vi "一体站流程质控自动启动.vi"(6 "CODMn量程切换":enum32{"H", "L", "AUTO"}(ring)=enum."AUTO", 8 "总磷量程切换":enum32{"H", "L", "AUTO"}(ring)=enum."AUTO", 9 "总氮量程切换":enum32{"H", "L", "AUTO"}(ring)=enum."AUTO", 10 "氨氮量程切换":enum32{"H", "L", "AUTO"}(ring)=enum."AUTO", 11 "参数":T1={"是否启用仪器"=FALSE, "CODMn"={"启动测量模式"={"测量模式"=enum."水样测量"}, "确定按钮"=TRUE}, "启动模块"={"氨氮"=FALSE, "总磷"=FALSE, "总氮"=FALSE, "CODMn"=FALSE, "CODCr"=FALSE}, "常规启动"=FALSE, "直接启动"=FALSE}) -> ()   [LabVIEW 2016, in "质控单元.lvlib"]
panel:
  out "枚举 2":enum16{"初始化", "采配水启动", "等待", "配水", "排水", "结束"}(ring)
  out "枚举":enum16{"初始化", "采配水启动", "等待", "配水", "排水", "结束"}(ring)
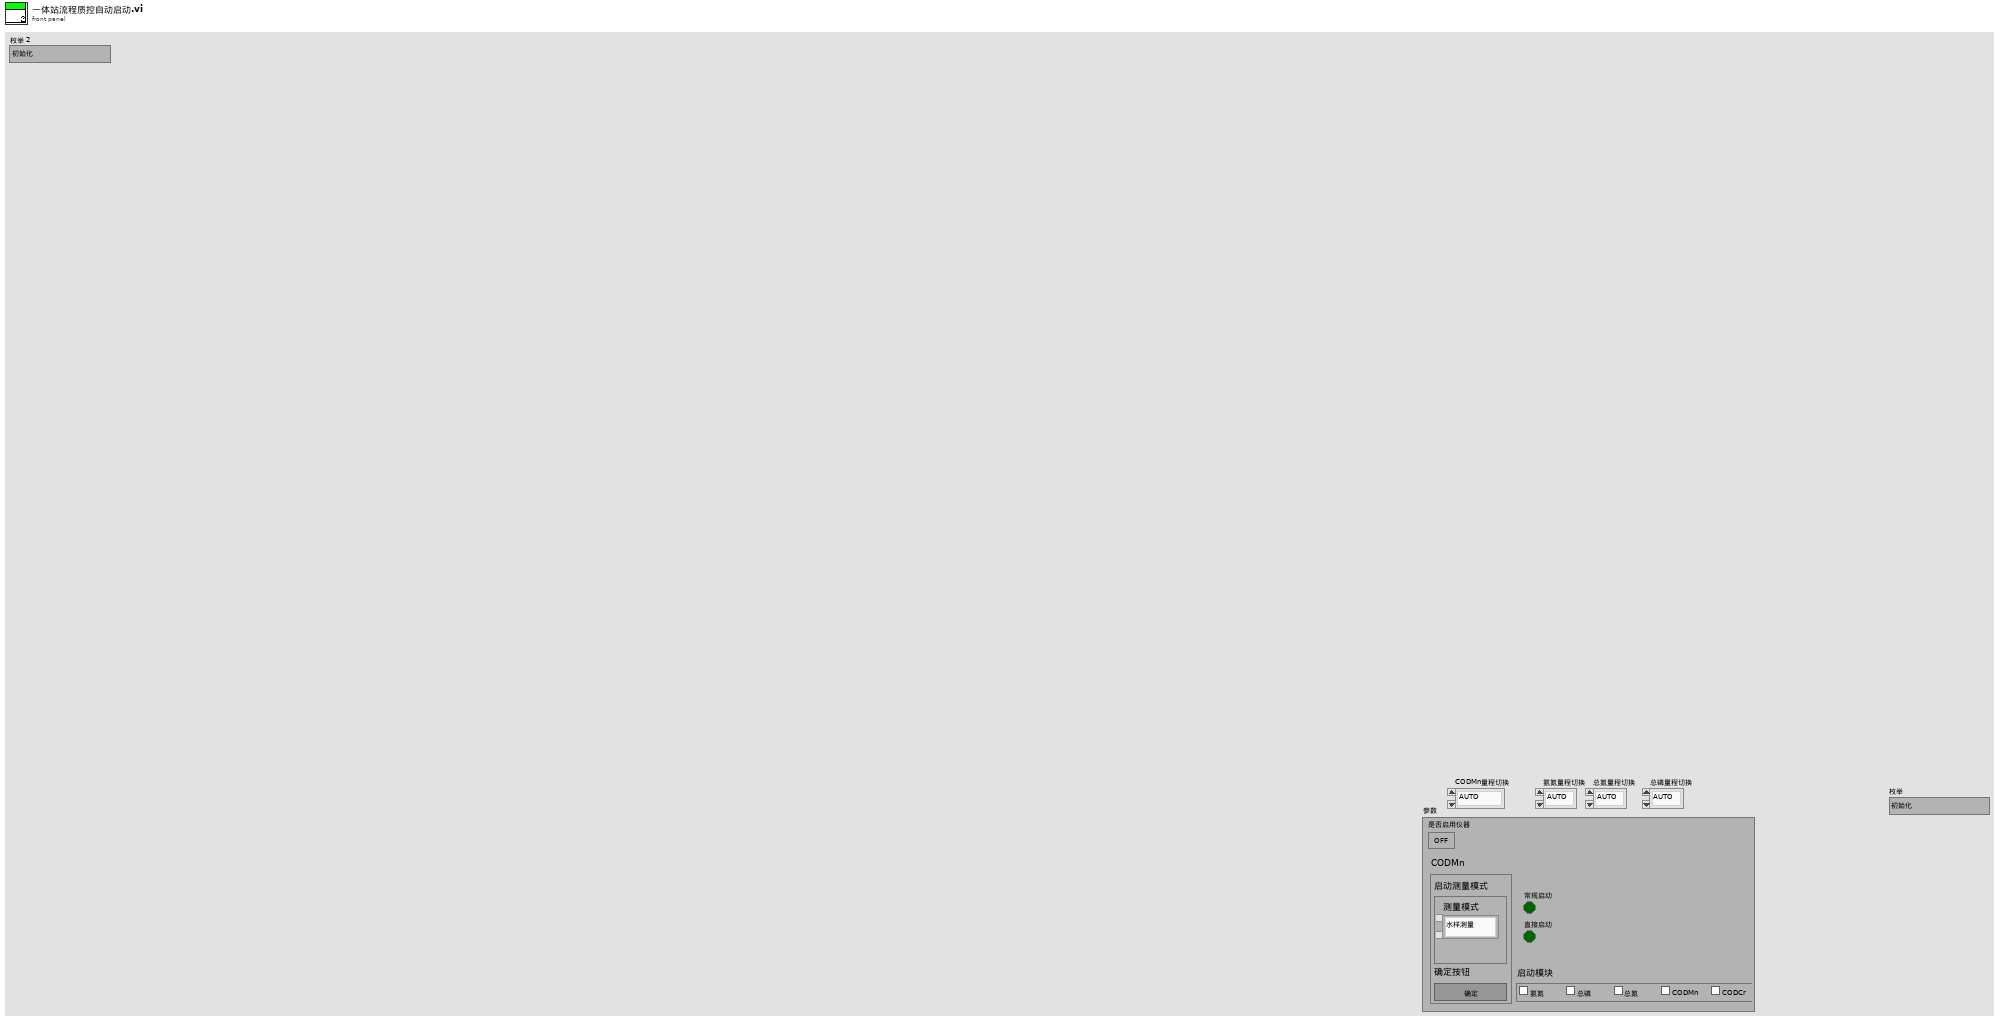
[diagram p1: front panel]
types:
  T1 = cluster{"是否启用仪器":bool, "CODMn":cluster{"启动测量模式":cluster{"测量模式":enum16{"水样测量", "标样核查", "加标回收", "平行样", "校零", "校标"}}, "确定按钮":bool}, "启动模块":cluster{"氨氮":bool, "总磷":bool, "总氮":bool, "CODMn":bool, "CODCr":bool}, "常规启动":bool, "直接启动":bool}
  T2 = cluster{"命令":string, cluster{"starting address":u16, "holding register value":u16}}
  T3 = cluster{"R0":i16, "R1":i16, "R2":i16, "R3":i16, "R4":i16, "R5":i16, "R6":i16, "R7":i16, "R8":i16, "R9":i16, "R10":i16, "R11":i16, "R12":i16, "R13":i16, "R14":i16, "R15":i16, "R16":i16, "R17":i16, "R18":i16, "R19":i16, "R20":i16, "R21":i16, "R22":i16, "R23":i16, "R24":i16, "R25":i16, "R26":i16, "R27":i16, "R28":i16, "R29":i16, "R30":i16, "R31":i16, "R32":i16, "R33":i16, "R34":i16, "R35":i16, "R36":i16, "R37":i16, "R38":i16, "R39":i16, "R40":i16, "R41":i16, "R42":i16, "R43":i16, "R44":i16, "R45":i16, "R46":i16, "R47":i16, "R48":i16, "R49":i16, "R50":i16, "R51":i16, "R52":i16, "R53":i16, "R54":i16, "R55":i16, "R56":i16}
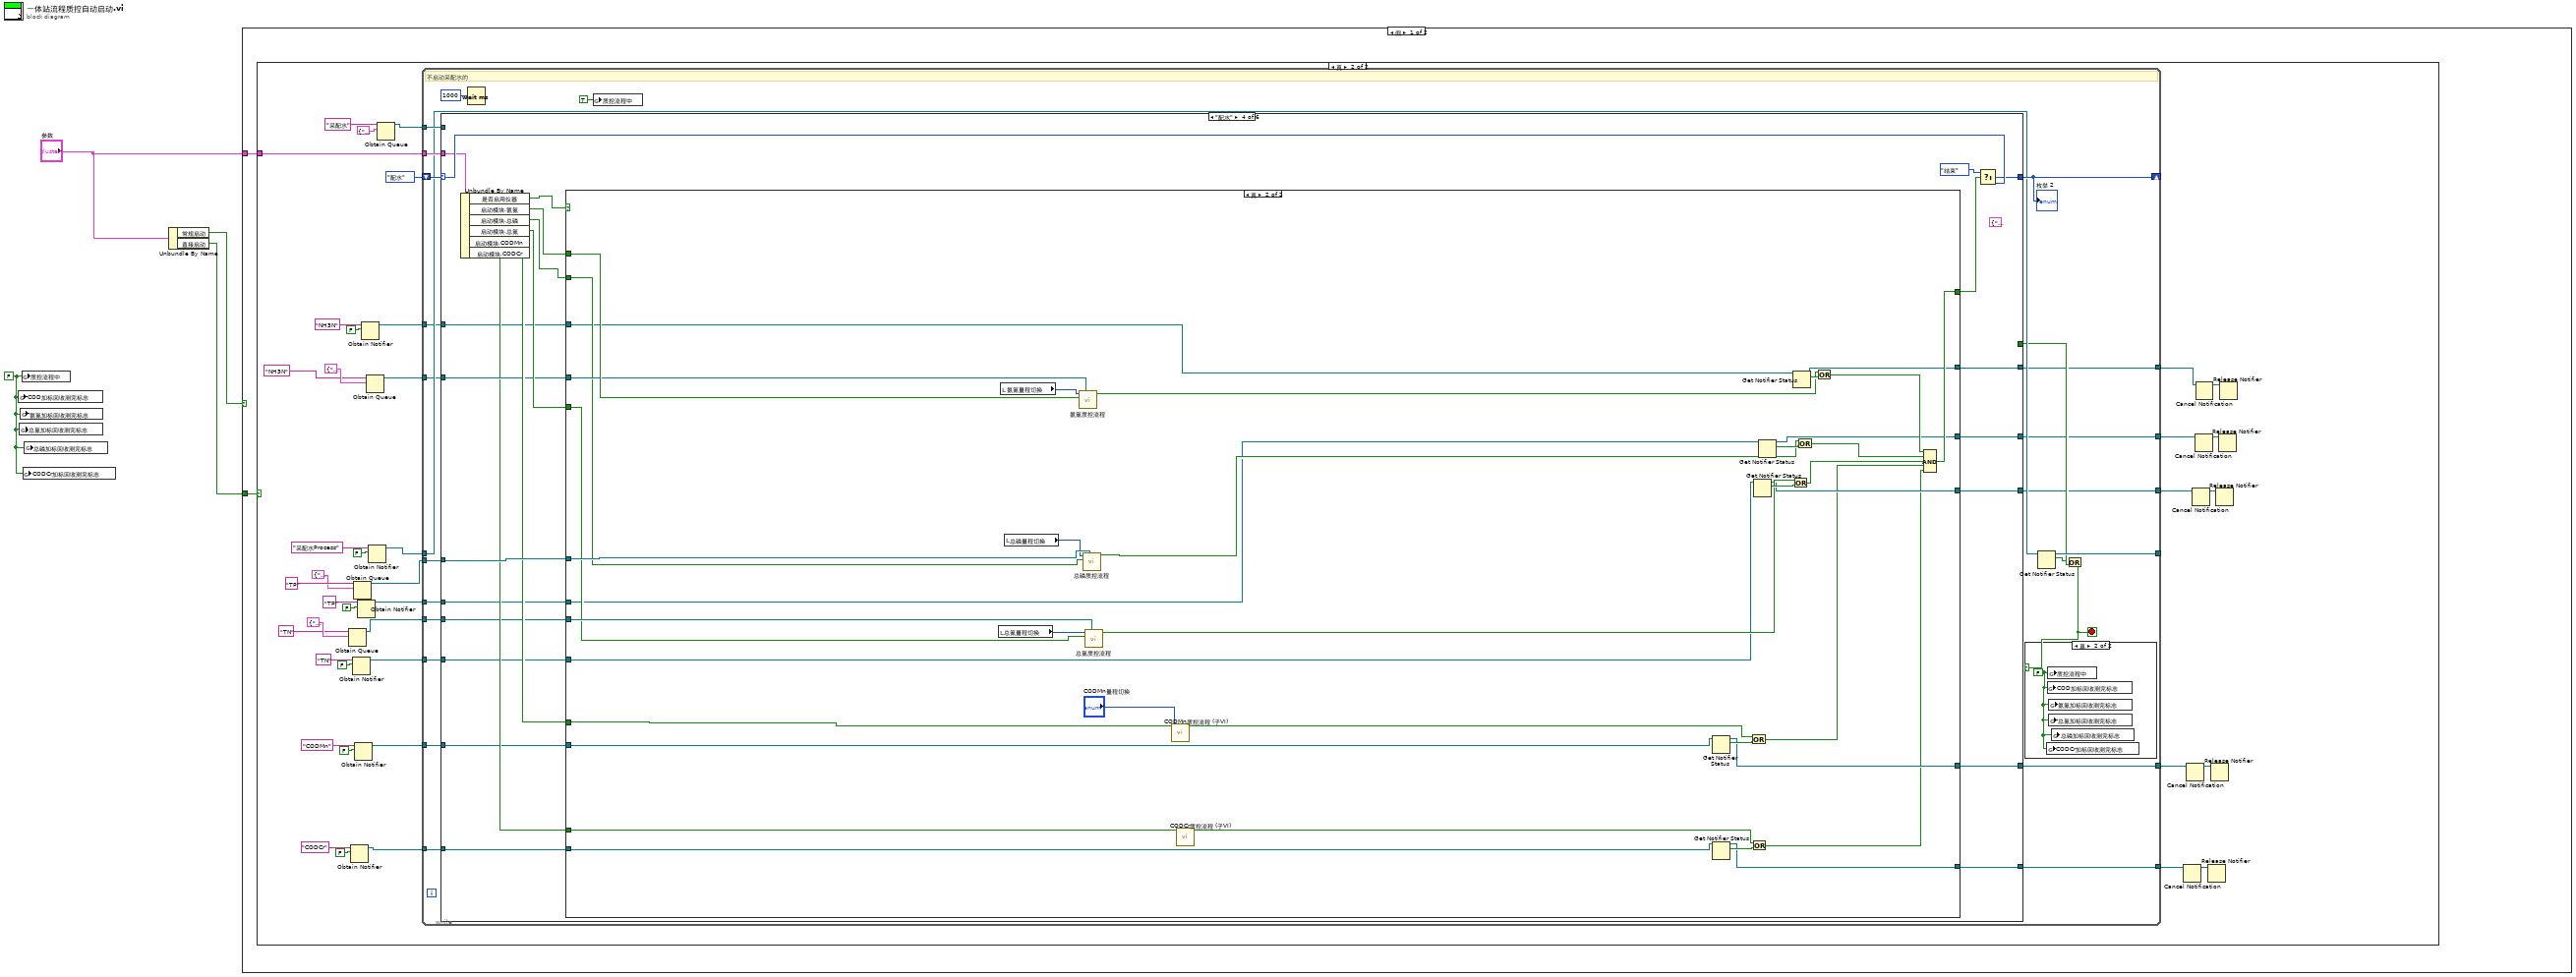
[diagram p0: block diagram]
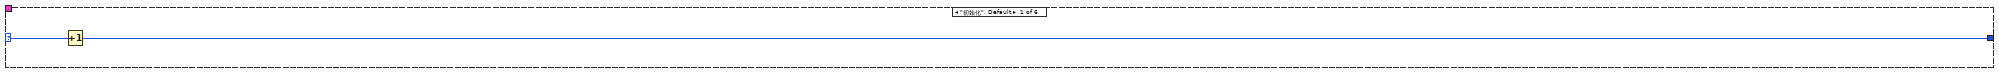
[diagram p4: hidden frame]
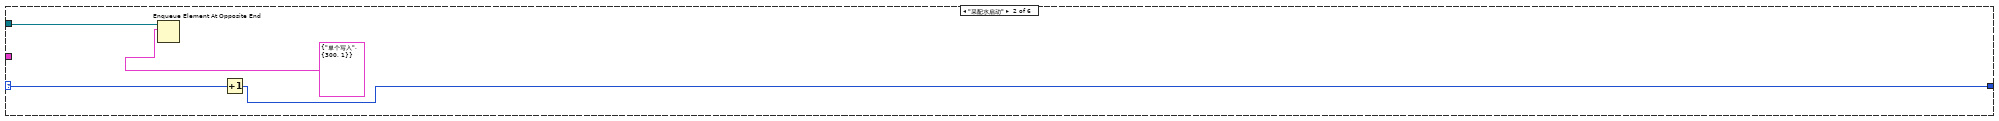
[diagram p5: hidden frame]
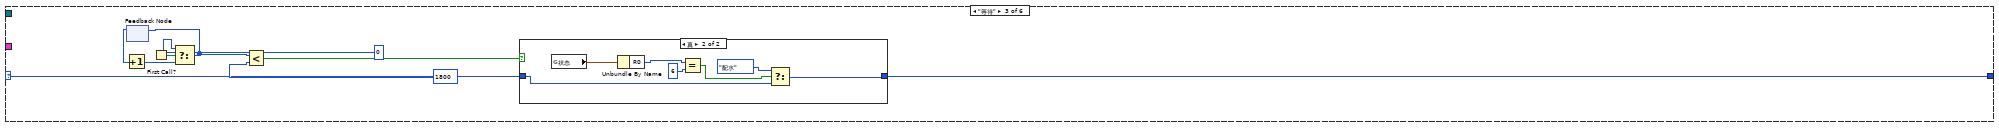
[diagram p6: hidden frame]
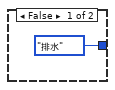
[diagram p7: hidden frame]
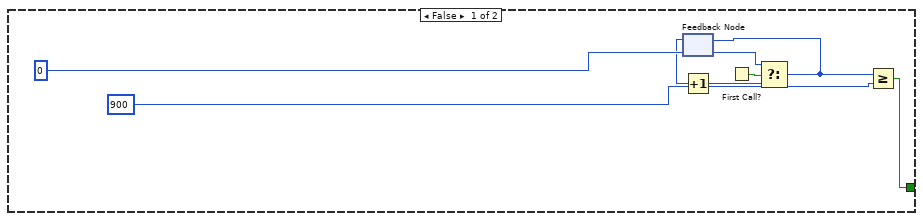
[diagram p8: hidden frame]
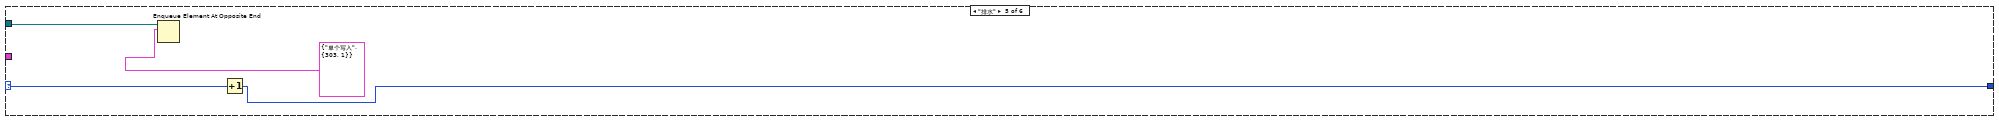
[diagram p9: hidden frame]
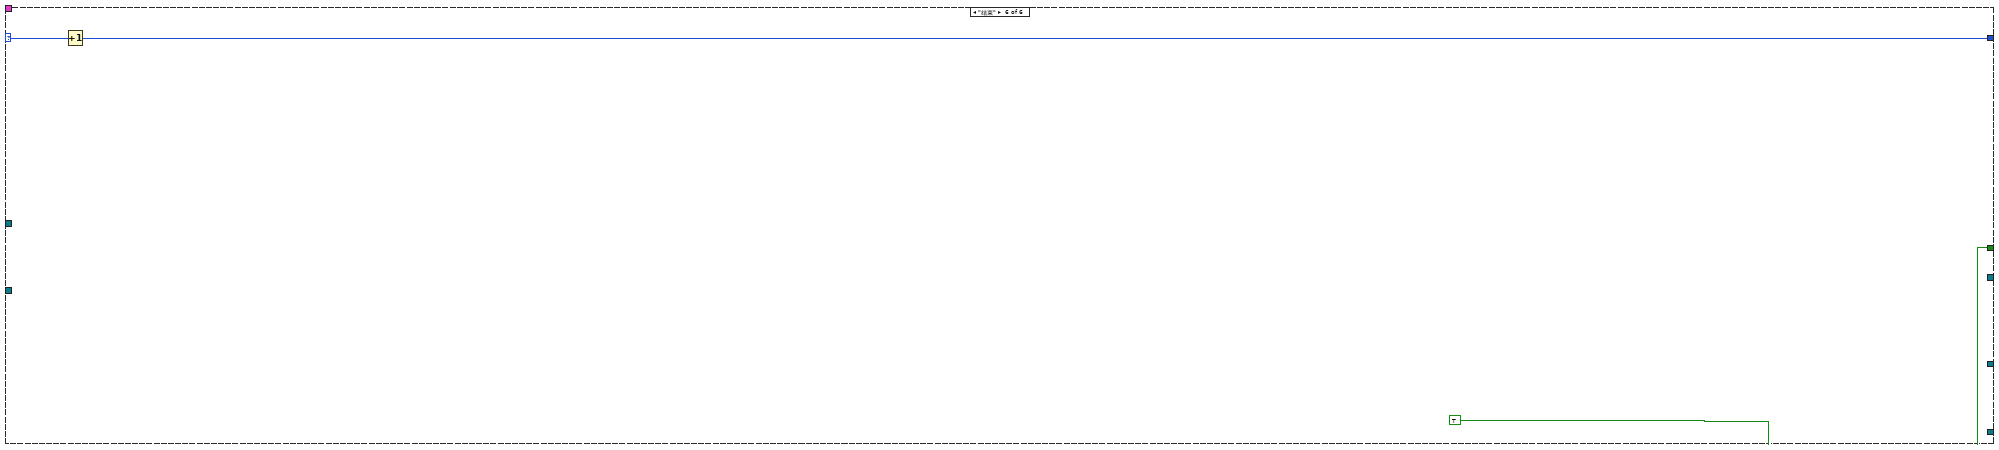
[diagram p10: hidden frame]
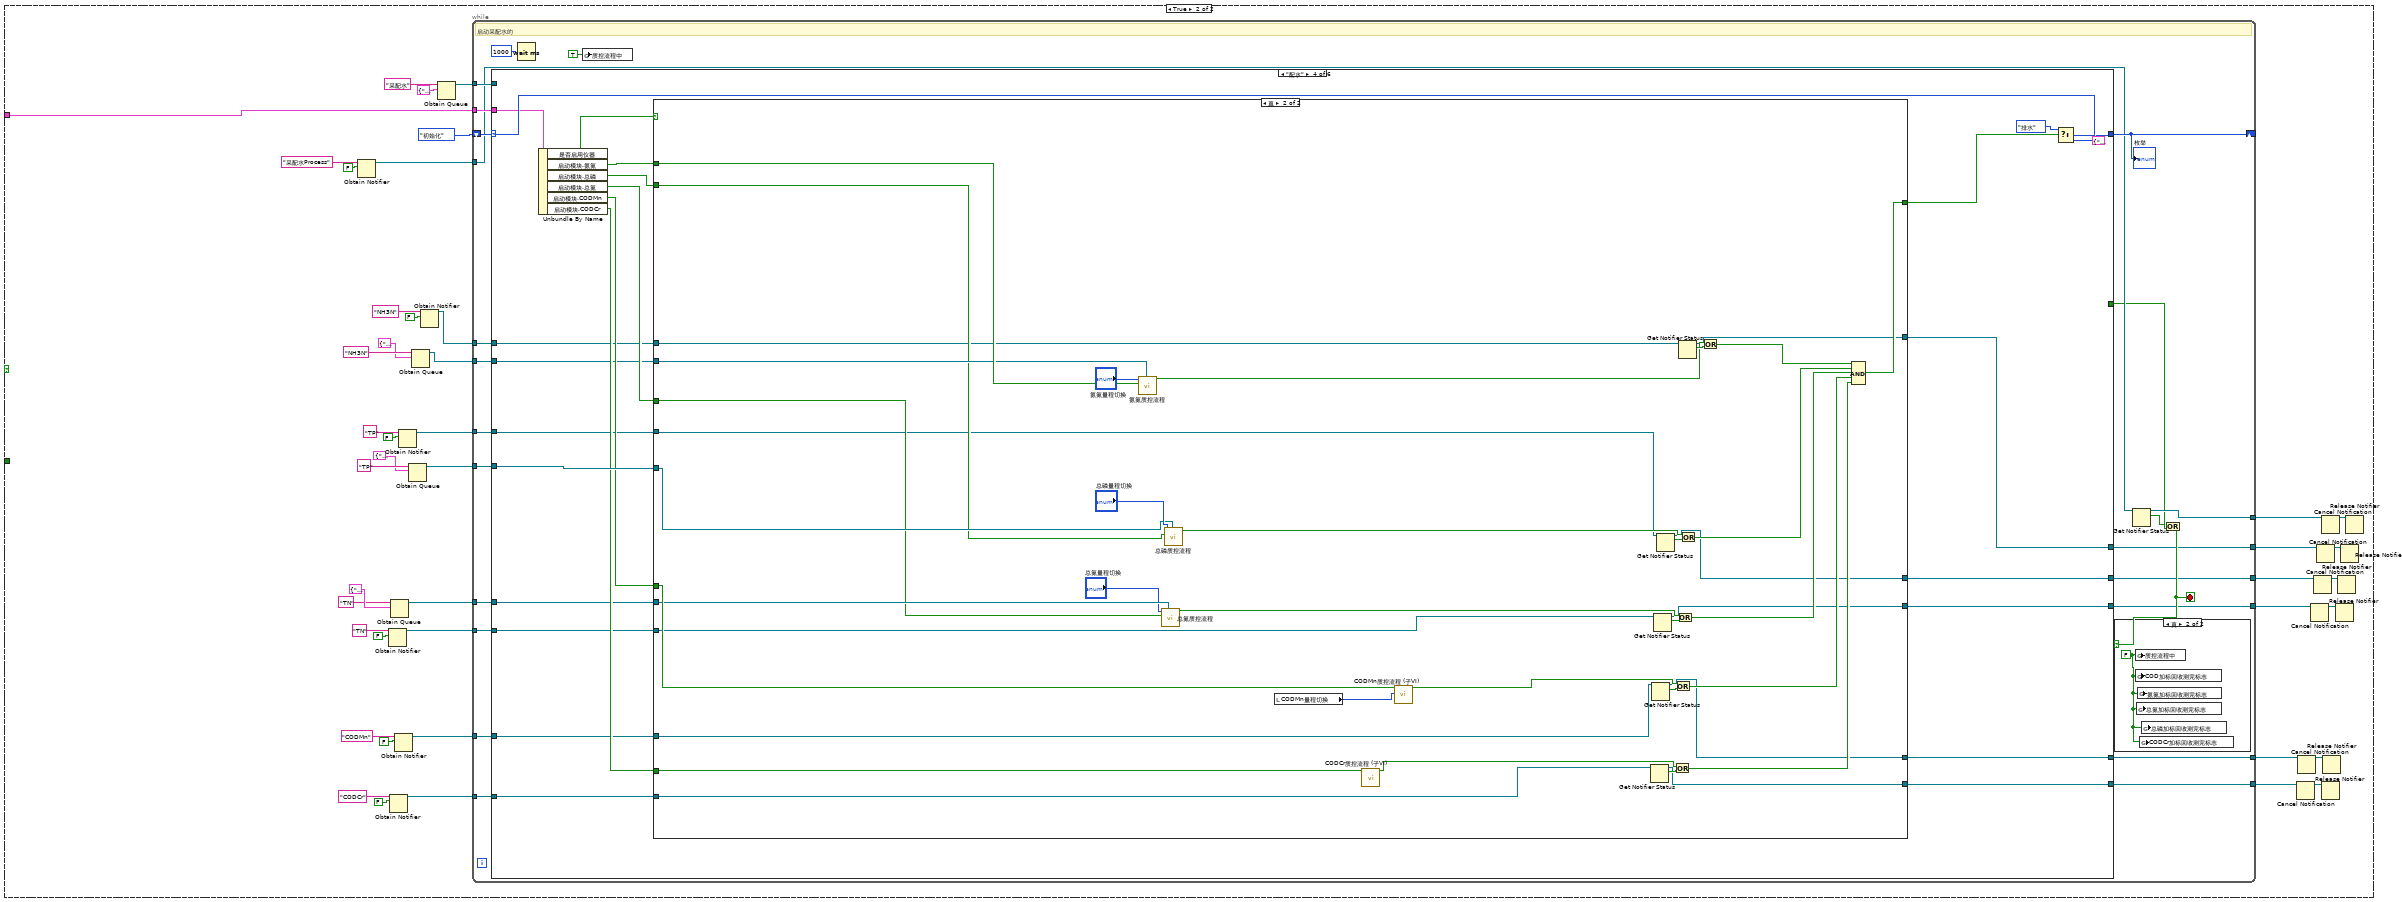
[diagram p11: hidden frame]
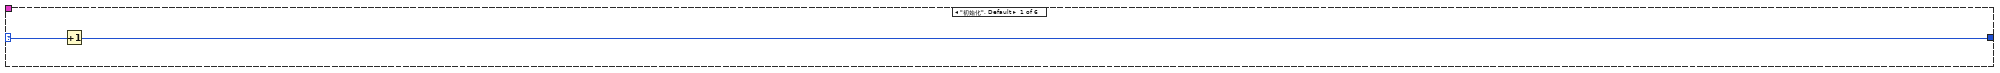
[diagram p13: hidden frame]
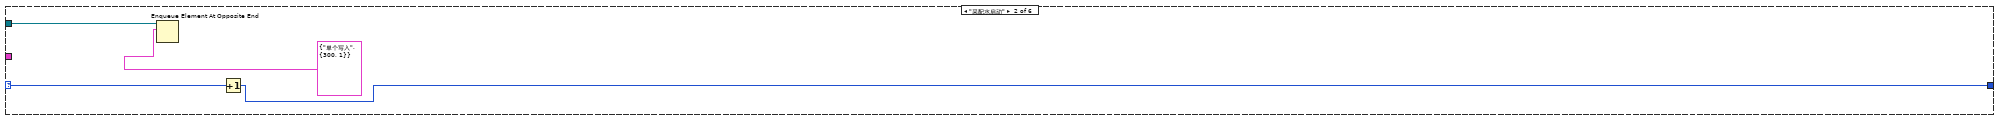
[diagram p14: hidden frame]
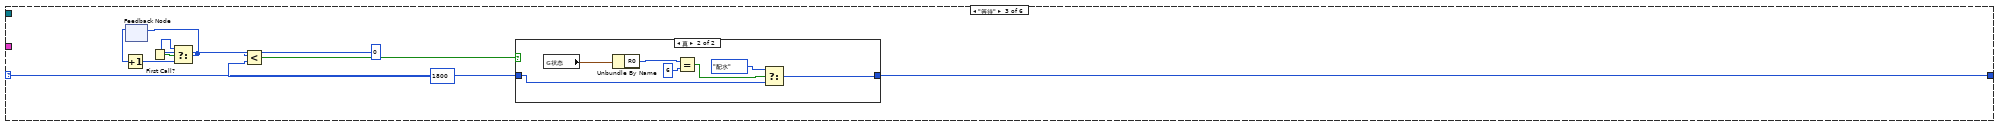
[diagram p15: hidden frame]
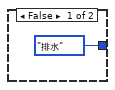
[diagram p16: hidden frame]
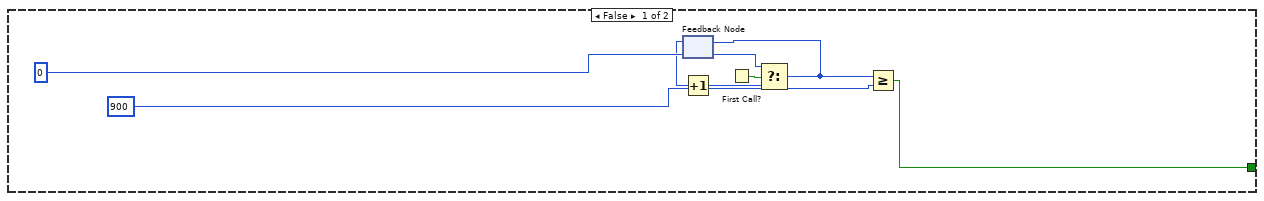
[diagram p17: hidden frame]
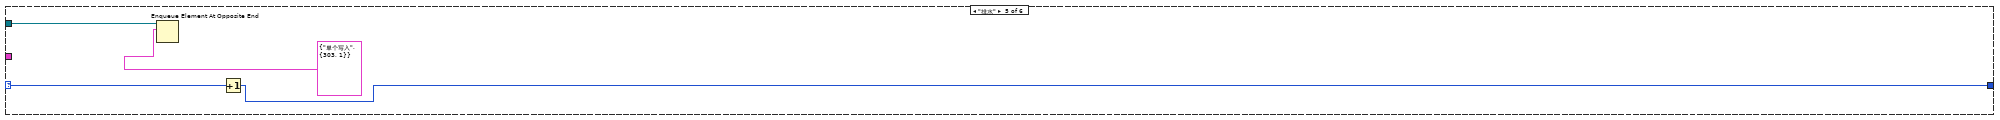
[diagram p18: hidden frame]
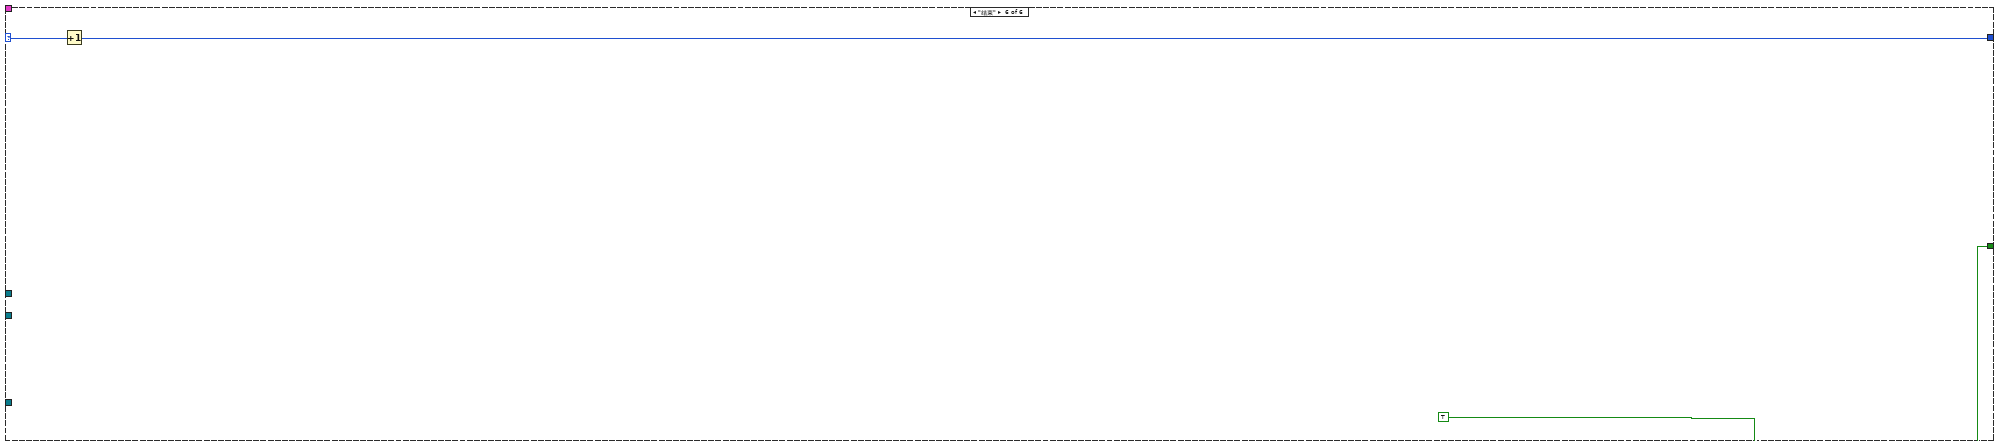
[diagram p19: hidden frame]
diagram:
  w1 = FALSE ("质控流程中")
  n1 = global write "质控测完标志全局 1.vi" "COD加标回收测完标志"(w1) -> ()
  n2 = global write "质控测完标志全局 1.vi" "总氮加标回收测完标志"(w1) -> ()
  n3 = global write "质控测完标志全局 1.vi" "氨氮加标回收测完标志"(w1) -> ()
  n4 = global write "质控测完标志全局 1.vi" "质控流程中"(w1) -> ()
  n5 = global write "质控测完标志全局 1.vi" "CODCr加标回收测完标志"(w1) -> ()
  n6 = global write "质控测完标志全局 1.vi" "总磷加标回收测完标志"(w1) -> ()
  n7 = Unbundle By Name("参数") -> ("常规启动"=w3:bool, "直接启动"=w2:bool)
  n8 = case shown="假" w3 {
    tunnel: "参数" -> [w5 w204]
    tunnel: w2 -> [w6 _]
    frame False {
      n9 = case shown="真" w6 {
        tunnel: w5 -> [_ w47]
        frame False {
        }
        frame True {
          n10 = Obtain Queue(name (unnamed)="TN" ("名称（未命名）"), element data type=cluster{"命令":string, "data":variant} {"命令"="", "data"=variant}) -> (queue out=w32:refnum<queue>)  [unwired: 3 in, 2 out]
          n11 = Obtain Notifier(name (unnamed)="CODCr" ("名称（未命名）"), notification data type=FALSE) -> (notifier out=w9:refnum<notifier>)  [unwired: 2 in, 2 out]
          n12 = Obtain Notifier(name (unnamed)="TN" ("名称（未命名）"), notification data type=FALSE) -> (notifier out=w15:refnum<notifier>)  [unwired: 2 in, 2 out]
          n13 = Obtain Queue(name (unnamed)="TP" ("名称（未命名）"), element data type=cluster{"命令":string, "data":variant} {"命令"="", "data"=variant}) -> (queue out=w38:refnum<queue>)  [unwired: 3 in, 2 out]
          n14 = Obtain Notifier(name (unnamed)="CODMn" ("名称（未命名）"), notification data type=FALSE) -> (notifier out=w12:refnum<notifier>)  [unwired: 2 in, 2 out]
          n15 = Obtain Notifier(name (unnamed)="TP" ("名称（未命名）"), notification data type=FALSE) -> (notifier out=w18:refnum<notifier>)  [unwired: 2 in, 2 out]
          n16 = Obtain Notifier(name (unnamed)="NH3N" ("名称（未命名）"), notification data type=FALSE) -> (notifier out=w21:refnum<notifier>)  [unwired: 2 in, 2 out]
          n17 = Obtain Queue(name (unnamed)="NH3N" ("名称（未命名）"), element data type=cluster{"命令":string, "data":variant} {"命令"="", "data"=variant}) -> (queue out=w35:refnum<queue>)  [unwired: 3 in, 2 out]
          n18 = Obtain Notifier(name (unnamed)="采配水Process" ("名称（未命名）"), notification data type=FALSE) -> (notifier out=w41:refnum<notifier>)  [unwired: 2 in, 2 out]
          n19 = Obtain Queue(name (unnamed)="采配水" ("名称（未命名）"), element data type=cluster{"命令":string, "数据":variant} {"命令"="", "数据"=variant}) -> (queue out=w44:refnum<queue>)  [unwired: 3 in, 2 out]
          n20 = while {
            tunnel: w44 -> [w72]
            shift-right: [w70] -> _
            shift-left: enum16{"初始化", "采配水启动", "等待", "配水", "排水", "结束"}."配水" ("枚举") -> [w71]
            tunnel: w38 -> [w68]
            tunnel: w47 -> [w67]
            tunnel: w41 -> [w66]
            tunnel: [w65] -> _
            tunnel: w35 -> [w62]
            tunnel: w32 -> [w59]
            tunnel: w21 -> [w58]
            tunnel: [w57] -> w19
            tunnel: w18 -> [w56]
            tunnel: [w55] -> w16
            tunnel: w15 -> [w54]
            tunnel: [w53] -> w13
            tunnel: w12 -> [w52]
            tunnel: [w51] -> w10
            tunnel: w9 -> [w50]
            tunnel: [w49] -> w7
            stop <- w61 stop-if-true
            # "不启动采配水的"
            n21 = case shown="\"配水\"" w71 {
              selector: w71 -> [w75 w77 w86 w119 w167 w172]
              tunnel: w72 -> [_ w78 _ _ w168 _]
              tunnel: [w74 w76 w85 w118 w166 w171] -> w70
              tunnel: [_ _ _ _ _ TRUE] -> w64
              tunnel: w68 -> [_ _ _ w117 _ _]
              tunnel: w67 -> [_ _ _ w114 _ _]
              tunnel: w62 -> [_ _ _ w109 _ _]
              tunnel: w59 -> [_ _ _ w107 _ _]
              tunnel: w58 -> [_ _ _ w106 _ _]
              tunnel: [_ _ _ w105 _ _] -> w57
              tunnel: w56 -> [_ _ _ w104 _ _]
              tunnel: [_ _ _ w103 _ _] -> w55
              tunnel: w54 -> [_ _ _ w102 _ _]
              tunnel: [_ _ _ w101 _ _] -> w53
              tunnel: w52 -> [_ _ _ w100 _ _]
              tunnel: [_ _ _ w99 _ _] -> w51
              tunnel: w50 -> [_ _ _ w98 _ _]
              tunnel: [_ _ _ w97 _ _] -> w49
              frame "初始化", Default {
                n22 = Increment(x=w75) -> (x+1=w74:enum16{"初始化", "采配水启动", "等待", "配水", "排水", "结束"})
              }
              frame "采配水启动" {
                n23 = Enqueue Element At Opposite End(queue=w78, element=T2 {"命令"="单个写入", {"starting address"=300, "holding register value"=1}} ("元素")) -> ()  [unwired: 2 in, 3 out]
                n24 = Increment(x=w77) -> (x+1=w76:enum16{"初始化", "采配水启动", "等待", "配水", "排水", "结束"})
              }
              frame "等待" {
                n25 = feedback #1() -> (w82:i32)  [unwired: 1 in]
                n26 = Increment(x=w82) -> (x+1=w81:i32)
                n27 = First Call?() -> (First Call?: T/F=w83:bool)
                n28 = Select(t=0, s=w83, f=w81) -> (s? t:f=w80:i32)
                n29 = feedback-in #1(w80) -> ()
                n30 = Less?(x=w80, y=1800) -> (x < y?=w87:bool)
                n31 = case shown="真" w87 {
                  tunnel: w86 -> [_ w92]
                  tunnel: [enum16{"初始化", "采配水启动", "等待", "配水", "排水", "结束"}."排水" ("枚举") w91] -> w85
                  frame False {
                  }
                  frame True {
                    n32 = global read "与采配水交互全局.vi" "状态"() -> (w90:T3)
                    n33 = Unbundle By Name(w90) -> ("R0"=w96:i16)
                    n34 = Equal?(x=w96, y=i16 6) -> (x = y?=w94:bool)
                    n35 = Select(t=enum16{"初始化", "采配水启动", "等待", "配水", "排水", "结束"}."配水" ("枚举"), s=w94, f=w92) -> (s? t:f=w91:enum16{"初始化", "采配水启动", "等待", "配水", "排水", "结束"})
                  }
                }
              }
              frame "配水" {
                (unwired) cluster{"命令":string, "data":variant} {"命令"="启动", "data"=variant(cluster{"站号":u16, "控制命令输出":u16[]} {"站号"=1, "控制命令输出"=[256, 0]})} ("元素")
                n36 = Unbundle By Name(w114) -> ("是否启用仪器"=w116:bool, "启动模块.氨氮"=w112:bool, "启动模块.总磷"=w113:bool, "启动模块.总氮"=w110:bool, "启动模块.CODMn"=w111:bool, "启动模块.CODCr"=w108:bool)
                n37 = case shown="真" w116 {
                  tunnel: w117 -> [_ w158]
                  tunnel: [w121 w165] -> w115
                  tunnel: w113 -> [_ w156]
                  tunnel: w112 -> [_ w164]
                  tunnel: w111 -> [_ w163]
                  tunnel: w110 -> [_ w153]
                  tunnel: w109 -> [_ w162]
                  tunnel: w108 -> [_ w159]
                  tunnel: w107 -> [_ w155]
                  tunnel: w106 -> [_ w149]
                  tunnel: [_ w148] -> w105
                  tunnel: w104 -> [_ w145]
                  tunnel: [_ w143] -> w103
                  tunnel: w102 -> [_ w140]
                  tunnel: [_ w138] -> w101
                  tunnel: w100 -> [_ w134]
                  tunnel: [_ w133] -> w99
                  tunnel: w98 -> [_ w129]
                  tunnel: [_ w128] -> w97
                  frame False {
                    n38 = feedback #2() -> (w125:i32)  [unwired: 1 in]
                    n39 = Increment(x=w125) -> (x+1=w124:i32)
                    n40 = First Call?() -> (First Call?: T/F=w126:bool)
                    n41 = Select(t=0, s=w126, f=w124) -> (s? t:f=w122:i32)
                    n42 = feedback-in #2(w122) -> ()
                    n43 = Greater Or Equal?(x=w122, y=900) -> (x >= y?=w121:bool)
                  }
                  frame True {
                    n44 = local read "总氮量程切换"() -> (w154:enum32{"H", "L", "AUTO"})
                    n45 = local read "氨氮量程切换"() -> (w160:enum32{"H", "L", "AUTO"})
                    n46 = local read "总磷量程切换"() -> (w157:enum32{"H", "L", "AUTO"})
                    n47 = call "氨氮质控流程.vi"("队列输入NH3"=w162, "氨氮"=w164, "氨氮量程切换"=w160) -> ("布尔"=w150:bool)  [unwired: 7 in]
                    n48 = call "总磷质控流程.vi"("队列输入TP"=w158, "总磷"=w156, "总磷量程切换"=w157) -> ("布尔"=w146:bool)  [unwired: 7 in]
                    n49 = call "总氮质控流程.vi"("队列输入TN"=w155, "总氮"=w153, "总氮量程切换"=w154) -> ("布尔"=w141:bool)  [unwired: 7 in]
                    n50 = call "CODMn质控流程 (子VI).vi"("CODMn量程切换"="CODMn量程切换", "CODMn"=w163) -> ("布尔"=w136:bool)  [unwired: 8 in]
                    n51 = call "CODCr质控流程 (子VI).vi"("CODCr"=w159) -> ("布尔"=w131:bool)  [unwired: 9 in]
                    n52 = Get Notifier Status(notifier=w134) -> (notifier out=w133:refnum<notifier>, current notification=w137:bool)  [unwired: 1 in, 3 out]
                    n53 = Get Notifier Status(notifier=w129) -> (notifier out=w128:refnum<notifier>, current notification=w132:bool)  [unwired: 1 in, 3 out]
                    n54 = Or(x=w136, y=w137) -> (x .or. y?=w135:bool)
                    n55 = Or(x=w131, y=w132) -> (x .or. y?=w130:bool)
                    n56 = Get Notifier Status(notifier=w140) -> (notifier out=w138:refnum<notifier>, current notification=w142:bool)  [unwired: 1 in, 3 out]
                    n57 = Get Notifier Status(notifier=w145) -> (notifier out=w143:refnum<notifier>, current notification=w147:bool)  [unwired: 1 in, 3 out]
                    n58 = Or(x=w141, y=w142) -> (x .or. y?=w139:bool)
                    n59 = Get Notifier Status(notifier=w149) -> (notifier out=w148:refnum<notifier>, current notification=w152:bool)  [unwired: 1 in, 3 out]
                    n60 = Or(x=w146, y=w147) -> (x .or. y?=w144:bool)
                    n61 = Or(x=w150, y=w152) -> (x .or. y?=w151:bool)
                    n62 = Compound Arithmetic op=AND ("复合运算")(w151, w144, w139, w135, w130) -> (w165:bool)
                  }
                }
                n63 = Select(t=enum16{"初始化", "采配水启动", "等待", "配水", "排水", "结束"}."结束" ("枚举"), s=w115, f=w119) -> (s? t:f=w118:enum16{"初始化", "采配水启动", "等待", "配水", "排水", "结束"})
              }
              frame "排水" {
                n64 = Enqueue Element At Opposite End(queue=w168, element=T2 {"命令"="单个写入", {"starting address"=303, "holding register value"=1}} ("元素")) -> ()  [unwired: 2 in, 3 out]
                n65 = Increment(x=w167) -> (x+1=w166:enum16{"初始化", "采配水启动", "等待", "配水", "排水", "结束"})
              }
              frame "结束" {
                n66 = Increment(x=w172) -> (x+1=w171:enum16{"初始化", "采配水启动", "等待", "配水", "排水", "结束"})
              }
            }
            "枚举 2" <- w70
            n67 = Wait (ms)(milliseconds to wait=u32 1000 ("等待时间（毫秒）")) -> ()  [unwired: 1 out]
            n68 = global write "质控测完标志全局 1.vi" "质控流程中"(TRUE ("质控流程中")) -> ()
            n69 = Get Notifier Status(notifier=w66) -> (notifier out=w65:refnum<notifier>, current notification=w63:bool)  [unwired: 1 in, 3 out]
            n70 = Or(x=w63, y=w64) -> (x .or. y?=w61:bool)
            n71 = case shown="真" w61 {
              frame False {
              }
              frame True {
                w73 = FALSE ("质控流程中")
                n72 = global write "质控测完标志全局 1.vi" "CODCr加标回收测完标志"(w73) -> ()
                n73 = global write "质控测完标志全局 1.vi" "COD加标回收测完标志"(w73) -> ()
                n74 = global write "质控测完标志全局 1.vi" "质控流程中"(w73) -> ()
                n75 = global write "质控测完标志全局 1.vi" "总氮加标回收测完标志"(w73) -> ()
                n76 = global write "质控测完标志全局 1.vi" "氨氮加标回收测完标志"(w73) -> ()
                n77 = global write "质控测完标志全局 1.vi" "总磷加标回收测完标志"(w73) -> ()
              }
            }
          }
          n78 = Cancel Notification(0:w7) -> (8:w8:refnum<notifier>)  [unwired: 1 in, 2 out]
          n79 = Cancel Notification(0:w10) -> (8:w11:refnum<notifier>)  [unwired: 1 in, 2 out]
          n80 = Cancel Notification(0:w13) -> (8:w14:refnum<notifier>)  [unwired: 1 in, 2 out]
          n81 = Cancel Notification(0:w16) -> (8:w17:refnum<notifier>)  [unwired: 1 in, 2 out]
          n82 = Cancel Notification(0:w19) -> (8:w20:refnum<notifier>)  [unwired: 1 in, 2 out]
          n83 = Release Notifier(notifier=w8) -> ()  [unwired: 2 in, 3 out]
          n84 = Release Notifier(notifier=w11) -> ()  [unwired: 2 in, 3 out]
          n85 = Release Notifier(notifier=w14) -> ()  [unwired: 2 in, 3 out]
          n86 = Release Notifier(notifier=w17) -> ()  [unwired: 2 in, 3 out]
          n87 = Release Notifier(notifier=w20) -> ()  [unwired: 2 in, 3 out]
        }
      }
    }
    frame True {
      n88 = Obtain Notifier(name (unnamed)="采配水Process" ("名称（未命名）"), notification data type=FALSE) -> (notifier out=w207:refnum<notifier>)  [unwired: 2 in, 2 out]
      n89 = Obtain Notifier(name (unnamed)="TN" ("名称（未命名）"), notification data type=FALSE) -> (notifier out=w189:refnum<notifier>)  [unwired: 2 in, 2 out]
      n90 = Obtain Notifier(name (unnamed)="CODCr" ("名称（未命名）"), notification data type=FALSE) -> (notifier out=w183:refnum<notifier>)  [unwired: 2 in, 2 out]
      n91 = Obtain Queue(name (unnamed)="TN" ("名称（未命名）"), element data type=cluster{"命令":string, "data":variant} {"命令"="", "data"=variant}) -> (queue out=w201:refnum<queue>)  [unwired: 3 in, 2 out]
      n92 = Obtain Notifier(name (unnamed)="CODMn" ("名称（未命名）"), notification data type=FALSE) -> (notifier out=w184:refnum<notifier>)  [unwired: 2 in, 2 out]
      n93 = Obtain Notifier(name (unnamed)="TP" ("名称（未命名）"), notification data type=FALSE) -> (notifier out=w190:refnum<notifier>)  [unwired: 2 in, 2 out]
      n94 = Obtain Queue(name (unnamed)="TP" ("名称（未命名）"), element data type=cluster{"命令":string, "data":variant} {"命令"="", "data"=variant}) -> (queue out=w210:refnum<queue>)  [unwired: 3 in, 2 out]
      n95 = Obtain Queue(name (unnamed)="NH3N" ("名称（未命名）"), element data type=cluster{"命令":string, "data":variant} {"命令"="", "data"=variant}) -> (queue out=w196:refnum<queue>)  [unwired: 3 in, 2 out]
      n96 = Obtain Notifier(name (unnamed)="NH3N" ("名称（未命名）"), notification data type=FALSE) -> (notifier out=w195:refnum<notifier>)  [unwired: 2 in, 2 out]
      n97 = Obtain Queue(name (unnamed)="采配水" ("名称（未命名）"), element data type=cluster{"命令":string, "数据":variant} {"命令"="", "数据"=variant}) -> (queue out=w214:refnum<queue>)  [unwired: 3 in, 2 out]
      n98 = while {
        tunnel: w214 -> [w240]
        shift-right: [w238] -> _
        shift-left: enum16{"初始化", "采配水启动", "等待", "配水", "排水", "结束"}."初始化" ("枚举") -> [w239]
        tunnel: w210 -> [w236]
        tunnel: w204 -> [w235]
        tunnel: w207 -> [w234]
        tunnel: [w233] -> w206
        tunnel: w201 -> [w228]
        tunnel: w196 -> [w227]
        tunnel: w195 -> [w226]
        tunnel: w190 -> [w225]
        tunnel: w189 -> [w224]
        tunnel: w184 -> [w223]
        tunnel: w183 -> [w222]
        tunnel: [w221] -> w181
        tunnel: [w220] -> w179
        tunnel: [w219] -> w177
        tunnel: [w218] -> w175
        tunnel: [w217] -> w173
        stop <- w230 stop-if-true
        # "启动采配水的"
        n99 = case shown="\"配水\"" w239 {
          selector: w239 -> [w243 w245 w254 w287 w335 w340]
          tunnel: w240 -> [_ w246 _ _ w336 _]
          tunnel: [w242 w244 w253 w286 w334 w339] -> w238
          tunnel: [_ _ _ _ _ TRUE] -> w232
          tunnel: w236 -> [_ _ _ w285 _ _]
          tunnel: w235 -> [_ _ _ w282 _ _]
          tunnel: w228 -> [_ _ _ w276 _ _]
          tunnel: w227 -> [_ _ _ w275 _ _]
          tunnel: w226 -> [_ _ _ w274 _ _]
          tunnel: w225 -> [_ _ _ w273 _ _]
          tunnel: w224 -> [_ _ _ w272 _ _]
          tunnel: w223 -> [_ _ _ w271 _ _]
          tunnel: w222 -> [_ _ _ w270 _ _]
          tunnel: [_ _ _ w269 _ _] -> w221
          tunnel: [_ _ _ w268 _ _] -> w220
          tunnel: [_ _ _ w267 _ _] -> w219
          tunnel: [_ _ _ w266 _ _] -> w218
          tunnel: [_ _ _ w265 _ _] -> w217
          frame "初始化", Default {
            n100 = Increment(x=w243) -> (x+1=w242:enum16{"初始化", "采配水启动", "等待", "配水", "排水", "结束"})
          }
          frame "采配水启动" {
            n101 = Enqueue Element At Opposite End(queue=w246, element=T2 {"命令"="单个写入", {"starting address"=300, "holding register value"=1}} ("元素")) -> ()  [unwired: 2 in, 3 out]
            n102 = Increment(x=w245) -> (x+1=w244:enum16{"初始化", "采配水启动", "等待", "配水", "排水", "结束"})
          }
          frame "等待" {
            n103 = feedback #3() -> (w250:i32)  [unwired: 1 in]
            n104 = Increment(x=w250) -> (x+1=w249:i32)
            n105 = First Call?() -> (First Call?: T/F=w251:bool)
            n106 = Select(t=0, s=w251, f=w249) -> (s? t:f=w248:i32)
            n107 = feedback-in #3(w248) -> ()
            n108 = Less?(x=w248, y=1800) -> (x < y?=w255:bool)
            n109 = case shown="真" w255 {
              tunnel: w254 -> [_ w260]
              tunnel: [enum16{"初始化", "采配水启动", "等待", "配水", "排水", "结束"}."排水" ("枚举") w259] -> w253
              frame False {
              }
              frame True {
                n110 = global read "与采配水交互全局.vi" "状态"() -> (w258:T3)
                n111 = Unbundle By Name(w258) -> ("R0"=w264:i16)
                n112 = Equal?(x=w264, y=i16 6) -> (x = y?=w262:bool)
                n113 = Select(t=enum16{"初始化", "采配水启动", "等待", "配水", "排水", "结束"}."配水" ("枚举"), s=w262, f=w260) -> (s? t:f=w259:enum16{"初始化", "采配水启动", "等待", "配水", "排水", "结束"})
              }
            }
          }
          frame "配水" {
            (unwired) cluster{"命令":string, "data":variant} {"命令"="启动", "data"=variant(cluster{"站号":u16, "控制命令输出":u16[]} {"站号"=1, "控制命令输出"=[256, 0]})} ("元素")
            n114 = Unbundle By Name(w282) -> ("是否启用仪器"=w284:bool, "启动模块.氨氮"=w280:bool, "启动模块.总磷"=w281:bool, "启动模块.总氮"=w278:bool, "启动模块.CODMn"=w279:bool, "启动模块.CODCr"=w277:bool)
            n115 = case shown="真" w284 {
              tunnel: w285 -> [_ w325]
              tunnel: [w289 w333] -> w283
              tunnel: w281 -> [_ w324]
              tunnel: w280 -> [_ w332]
              tunnel: w279 -> [_ w331]
              tunnel: w278 -> [_ w321]
              tunnel: w275 -> [_ w330]
              tunnel: w277 -> [_ w327]
              tunnel: w276 -> [_ w323]
              tunnel: w274 -> [_ w317]
              tunnel: w273 -> [_ w313]
              tunnel: w272 -> [_ w310]
              tunnel: w271 -> [_ w302]
              tunnel: w270 -> [_ w301]
              tunnel: [_ w300] -> w269
              tunnel: [_ w299] -> w268
              tunnel: [_ w298] -> w267
              tunnel: [_ w297] -> w266
              tunnel: [_ w296] -> w265
              frame False {
                n116 = feedback #4() -> (w293:i32)  [unwired: 1 in]
                n117 = Increment(x=w293) -> (x+1=w292:i32)
                n118 = First Call?() -> (First Call?: T/F=w294:bool)
                n119 = Select(t=0, s=w294, f=w292) -> (s? t:f=w290:i32)
                n120 = feedback-in #4(w290) -> ()
                n121 = Greater Or Equal?(x=w290, y=900) -> (x >= y?=w289:bool)
              }
              frame True {
                n122 = call "氨氮质控流程.vi"("队列输入NH3"=w330, "氨氮"=w332, "氨氮量程切换"="氨氮量程切换") -> ("布尔"=w318:bool)  [unwired: 7 in]
                n123 = call "总氮质控流程.vi"("队列输入TN"=w323, "总氮"=w321, "总氮量程切换"="总氮量程切换") -> ("布尔"=w311:bool)  [unwired: 7 in]
                n124 = call "总磷质控流程.vi"("队列输入TP"=w325, "总磷"=w324, "总磷量程切换"="总磷量程切换") -> ("布尔"=w315:bool)  [unwired: 7 in]
                n125 = local read "CODMn量程切换"() -> (w329:enum32{"H", "L", "AUTO"})
                n126 = call "CODCr质控流程 (子VI).vi"("CODCr"=w327) -> ("布尔"=w303:bool)  [unwired: 9 in]
                n127 = call "CODMn质控流程 (子VI).vi"("CODMn量程切换"=w329, "CODMn"=w331) -> ("布尔"=w304:bool)  [unwired: 8 in]
                n128 = Get Notifier Status(notifier=w301) -> (notifier out=w296:refnum<notifier>, current notification=w307:bool)  [unwired: 1 in, 3 out]
                n129 = Get Notifier Status(notifier=w302) -> (notifier out=w297:refnum<notifier>, current notification=w308:bool)  [unwired: 1 in, 3 out]
                n130 = Get Notifier Status(notifier=w310) -> (notifier out=w298:refnum<notifier>, current notification=w312:bool)  [unwired: 1 in, 3 out]
                n131 = Get Notifier Status(notifier=w313) -> (notifier out=w299:refnum<notifier>, current notification=w316:bool)  [unwired: 1 in, 3 out]
                n132 = Or(x=w303, y=w307) -> (x .or. y?=w305:bool)
                n133 = Or(x=w304, y=w308) -> (x .or. y?=w306:bool)
                n134 = Or(x=w311, y=w312) -> (x .or. y?=w309:bool)
                n135 = Get Notifier Status(notifier=w317) -> (notifier out=w300:refnum<notifier>, current notification=w320:bool)  [unwired: 1 in, 3 out]
                n136 = Or(x=w315, y=w316) -> (x .or. y?=w314:bool)
                n137 = Or(x=w318, y=w320) -> (x .or. y?=w319:bool)
                n138 = Compound Arithmetic op=AND ("复合运算")(w319, w314, w309, w306, w305) -> (w333:bool)
              }
            }
            n139 = Select(t=enum16{"初始化", "采配水启动", "等待", "配水", "排水", "结束"}."排水" ("枚举"), s=w283, f=w287) -> (s? t:f=w286:enum16{"初始化", "采配水启动", "等待", "配水", "排水", "结束"})
          }
          frame "排水" {
            n140 = Enqueue Element At Opposite End(queue=w336, element=T2 {"命令"="单个写入", {"starting address"=303, "holding register value"=1}} ("元素")) -> ()  [unwired: 2 in, 3 out]
            n141 = Increment(x=w335) -> (x+1=w334:enum16{"初始化", "采配水启动", "等待", "配水", "排水", "结束"})
          }
          frame "结束" {
            n142 = Increment(x=w340) -> (x+1=w339:enum16{"初始化", "采配水启动", "等待", "配水", "排水", "结束"})
          }
        }
        "枚举" <- w238
        n143 = Wait (ms)(milliseconds to wait=u32 1000 ("等待时间（毫秒）")) -> ()  [unwired: 1 out]
        n144 = global write "质控测完标志全局 1.vi" "质控流程中"(TRUE ("质控流程中")) -> ()
        n145 = Get Notifier Status(notifier=w234) -> (notifier out=w233:refnum<notifier>, current notification=w231:bool)  [unwired: 1 in, 3 out]
        n146 = Or(x=w231, y=w232) -> (x .or. y?=w230:bool)
        n147 = case shown="真" w230 {
          frame False {
          }
          frame True {
            w241 = FALSE ("质控流程中")
            n148 = global write "质控测完标志全局 1.vi" "质控流程中"(w241) -> ()
            n149 = global write "质控测完标志全局 1.vi" "COD加标回收测完标志"(w241) -> ()
            n150 = global write "质控测完标志全局 1.vi" "总氮加标回收测完标志"(w241) -> ()
            n151 = global write "质控测完标志全局 1.vi" "氨氮加标回收测完标志"(w241) -> ()
            n152 = global write "质控测完标志全局 1.vi" "CODCr加标回收测完标志"(w241) -> ()
            n153 = global write "质控测完标志全局 1.vi" "总磷加标回收测完标志"(w241) -> ()
          }
        }
      }
      n154 = Cancel Notification(0:w173) -> (8:w174:refnum<notifier>)  [unwired: 1 in, 2 out]
      n155 = Cancel Notification(0:w175) -> (8:w176:refnum<notifier>)  [unwired: 1 in, 2 out]
      n156 = Cancel Notification(0:w177) -> (8:w178:refnum<notifier>)  [unwired: 1 in, 2 out]
      n157 = Cancel Notification(0:w179) -> (8:w180:refnum<notifier>)  [unwired: 1 in, 2 out]
      n158 = Cancel Notification(0:w181) -> (8:w182:refnum<notifier>)  [unwired: 1 in, 2 out]
      n159 = Cancel Notification(0:w206) -> (8:w205:refnum<notifier>)  [unwired: 1 in, 2 out]
      n160 = Release Notifier(notifier=w174) -> ()  [unwired: 2 in, 3 out]
      n161 = Release Notifier(notifier=w176) -> ()  [unwired: 2 in, 3 out]
      n162 = Release Notifier(notifier=w178) -> ()  [unwired: 2 in, 3 out]
      n163 = Release Notifier(notifier=w180) -> ()  [unwired: 2 in, 3 out]
      n164 = Release Notifier(notifier=w182) -> ()  [unwired: 2 in, 3 out]
      n165 = Release Notifier(notifier=w205) -> ()  [unwired: 2 in, 3 out]
    }
  }
